vi "Dashboard Main.vi"() -> ()   [LabVIEW 2012]
uses:
  <vilib>/event_ctls.llb/eventvkey.ctl
  <vilib>/Utility/config.llb/Read Key (String).vi
  <vilib>/Utility/config.llb/Read Key (I32).vi
  <vilib>/Utility/config.llb/Write Key (String).vi
  <vilib>/Utility/config.llb/Write Key (I32).vi
  <vilib>/Utility/config.llb/NI_LVConfig.lvlib
panel:
  out "Battery Value":dbl(slide) scale=0.0..14.0 scale format="%#_2e"
  out "Battery":sgl(graph)
  in  "Camera Settings":T1={"Frate Rate"=30, "Compression"=30, "Size"=1} {"Frate Rate" scale=1.0..30.0; "Size" items=["640x480", "320x240", "160x120"]}
  out "Mode":T2(ring)=enum."Auto Disabled"
  out "Camera IP":string
  out "JS1 Z":dbl(slide) scale=-1.0..1.0 scale format="%#_2e"
  out "JS2 Z":dbl(slide) scale=-1.0..1.0 scale format="%#_2e"
  out "Joystick 1":cluster{"X":dbl, "Y":dbl}[](graph)
  out "Joystick 2":cluster{"X":dbl, "Y":dbl}[](graph)
  out "JS Buttons 1":T3
  out "JS Buttons 2":T3
  out "MotorSlide4":dbl(slide) scale=-1.0..1.0 scale format="%#_2e"
  out "MotorSlide3":dbl(slide) scale=-1.0..1.0 scale format="%#_2e"
  out "MotorSlide2":dbl(slide) scale=-1.0..1.0 scale format="%#_2e"
  out "MotorName3":string="Front Left"
  out "MotorName4":string="Front Right"
  out "MotorName1":string="Rear Left"
  out "MotorName2":string="Rear Right"
  out "MotorChart4":dbl(graph)
  out "MotorChart3":dbl(graph)
  out "MotorChart2":dbl(graph)
  out "MotorSlide1":dbl(slide) scale=-1.0..1.0 scale format="%#_2e"
  out "MotorChart1":dbl(graph)
  out "Robot IP":string
  in  "Dashboard Tab":T4(tab)
  in  "Disable Autonomous":bool
  out "Arm Hook Sensor":bool
  out "Arm Encoder":dbl(knob) scale=0.0..100.0
  in  "notes":string
  out "Right Hook Sensor":bool
  out "Left Hook Sensor":bool
  out "Encoder Set":bool
  out "Arm Limit":bool
  in  "Dev Notes":string
  in  "Robot Subsystems":enum32{"Drive", "Arm", "Sensors", "Hotkeys"}(tab)
  in  "X-Throttle":dbl(slide)=1.0 min=0.0 max=1.0 step=0.1 scale=0.0..1.0
  in  "Y-Throttle":dbl(slide)=1.0 min=0.0 max=1.0 step=0.1 scale=0.0..1.0
  out "Left Wheel Encoder":dbl
  out "Right Wheel Encoder":dbl
  in  "Override Limit":bool
  out "Right Ultrasonic PWM":dbl(slide) scale=0.0..100.0
  out "Gyro":dbl(knob) scale=-180.0..180.0
  out "Left Ultrasonic PWM":dbl(slide) scale=0.0..100.0
  out "Hotkey Step":dbl
  out "Arm Preset":dbl
  in  "Current Hotkey":string
  out "Hotkey Running?":bool
  in  "Sim":bool=TRUE
  in  "Slider":dbl(slide) scale=0.0..100.0 scale format="%#_3g"
  in  "On/Off":bool caption="Solenoid"
  in  "Test Name":u16(ring) items=["Select the test to run...", "Example Test", "-------------------------------", "List of tests is built in robot code.", "Replace with your own automated tests."]
  in  "Test Tree":string(tree)
  in  "Motor":cluster{"Value":dbl, "Enable":bool} {"Value" scale=-1.0..1.0 scale format="%#_3g"}
  out "Progress":T5 {"Test Progress" scale=0.0..100.0}
  in  "Rev/Fwd":cluster{"Forward":bool, "Reverse":bool}
  in  "Ring":u16(ring) items=["Auto", "Fixed indoor", "Fixed outdoor 1", "Fixed outdoor 2", "Fixed fluorescent 1", "Fixed fluorescent 2", "Hold current"]
  in  "Listbox":i32(listbox)
  in  "Viewer":T6(tab)
  out "Mbps":dbl format="%#.1g"
  in  "Enable":bool
  in  "DB Camera Config":bool
  out "Mbps":bool
  out "fps":dbl format="%#.1g"
  out "Image Error Message":string="Timeout in Camera Communications"
  out "Camera Image":T7(plugin-control)
  out "Buttons 1":cluster{"1":bool, "2":bool, "3":bool}
  out "Kinect 1":cluster{"X":dbl, "Y":dbl, "Z":dbl} {"X" scale=1.0..-1.0; "Y" scale=1.0..-1.0; "Z" scale=1.0..-1.0}
  out "Buttons 2":cluster{"1":bool, "2":bool, "3":bool}
  out "Kinect 2":cluster{"X":dbl, "Y":dbl, "Z":dbl} {"X" scale=1.0..-1.0; "Y" scale=1.0..-1.0; "Z" scale=1.0..-1.0}
  out "Version":string
  out "Skeleton Picture":picture
  out "Players":i8
  out "Tree":string(tree)
  # "Drive & Motors"
  # "Robot IP:"
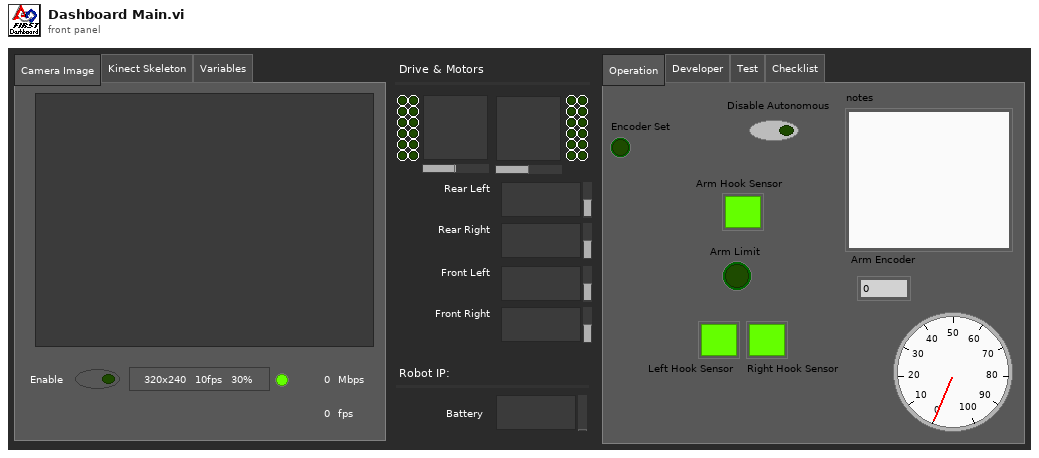
[diagram p1: front panel]
types:
  T1 = cluster{"Frate Rate":i32, "Compression":i32, "Size":u16}
  T2 = enum8{"Tele-Op Disabled", "Tele-Op Enabled", "Auto Disabled", "Auto Enabled", "Test Disabled", "Test Enabled", ""}
  T3 = cluster{bool, bool, bool, bool, bool, bool, bool, bool, bool, bool, bool, bool}
  T4 = enum32{"Operation", "Developer", "Test", "Checklist"}
  T5 = cluster{"Test Progress":u8, "Test Progress Text":string}
  T6 = enum32{"Camera Image", "Kinect Skeleton", "Variables"}
  T7 = typedef "IMAQ Image.ctl" = refnum<image>
  T8 = typedef "Image Type" = u32
  T9 = typedef "LVBoundsTypeDef.ctl" = cluster{"Width":u32, "Height":u32}
  T10 = typedef "SkeletonTrackState.ctl" = enum32{"NotTracked", "PositionOnly", "Tracked"}
  T11 = cluster{"TrackingState":u8[], "Position":cluster{"x":sgl, "y":sgl, "z":sgl}, cluster{"x":sgl, "y":sgl, "z":sgl, sgl}[], "TrackState":T10}
  T12 = cluster{cluster{"ScaledToPercentRange":dbl, "ScaledToPercentRange":dbl, "ScaledToPercentRange":dbl}, cluster{bool, bool, bool}}[]
  T13 = cluster{cluster{"ScaledToPercentRange":dbl, "ScaledToPercentRange":dbl, "ScaledToPercentRange":dbl}, cluster{bool, bool, bool}}
  T14 = cluster{"ScaledToPercentRange":dbl, "ScaledToPercentRange":dbl, "ScaledToPercentRange":dbl}
  T15 = typedef "LVRectTypeDef.ctl" = cluster{"Left":i16, "Top":i16, "Right":i16, "Bottom":i16}
  T16 = cluster{"Competition mode":bool, "Robot Link":bool, "Autonomous":bool, "Enabled":bool, "E-Stop":bool, "Simulated":bool, "TestMode":bool, "Docked Window":bool}
  T17 = cluster{"Boolean Array[0]":bool, "Boolean Array[1]":bool, "Boolean Array[2]":bool, "Boolean Array[3]":bool, "Boolean Array[4]":bool, "Boolean Array[5]":bool, "Boolean Array[6]":bool, "Boolean Array[7]":bool, "Boolean Array[8]":bool, "Boolean Array[9]":bool, "Boolean Array[10]":bool, "Boolean Array[11]":bool}
  T18 = typedef "NI_LVConfig.lvlib/Config Data RefNum.ctl" = refnum<k1>
  T19 = typedef "eventvkey.ctl" = enum16{"ASCII", "Enter", "Return", "Shift", "Ctrl", "Alt", "Cmd", "Opt", "Caps", "NumLock", "Clear", "Break", "Up", "Down", "Left", "Right", "Insert", "Delete", "Home", "End", "PageUp", "PageDown", "Escape", "Help", "Pause", "ScrollLock", "F1", "F2", "F3", "F4", "F5", "F6", "F7", "F8", "F9", "F10", "F11", "F12", "F13", "F14", "F15", "F16", "F17", "F18", "F19", "F20", "F21", "F22", "F23", "F24", "Play", "VolumeUp", "VolumeDown", "Mute", "Two Byte Char"}
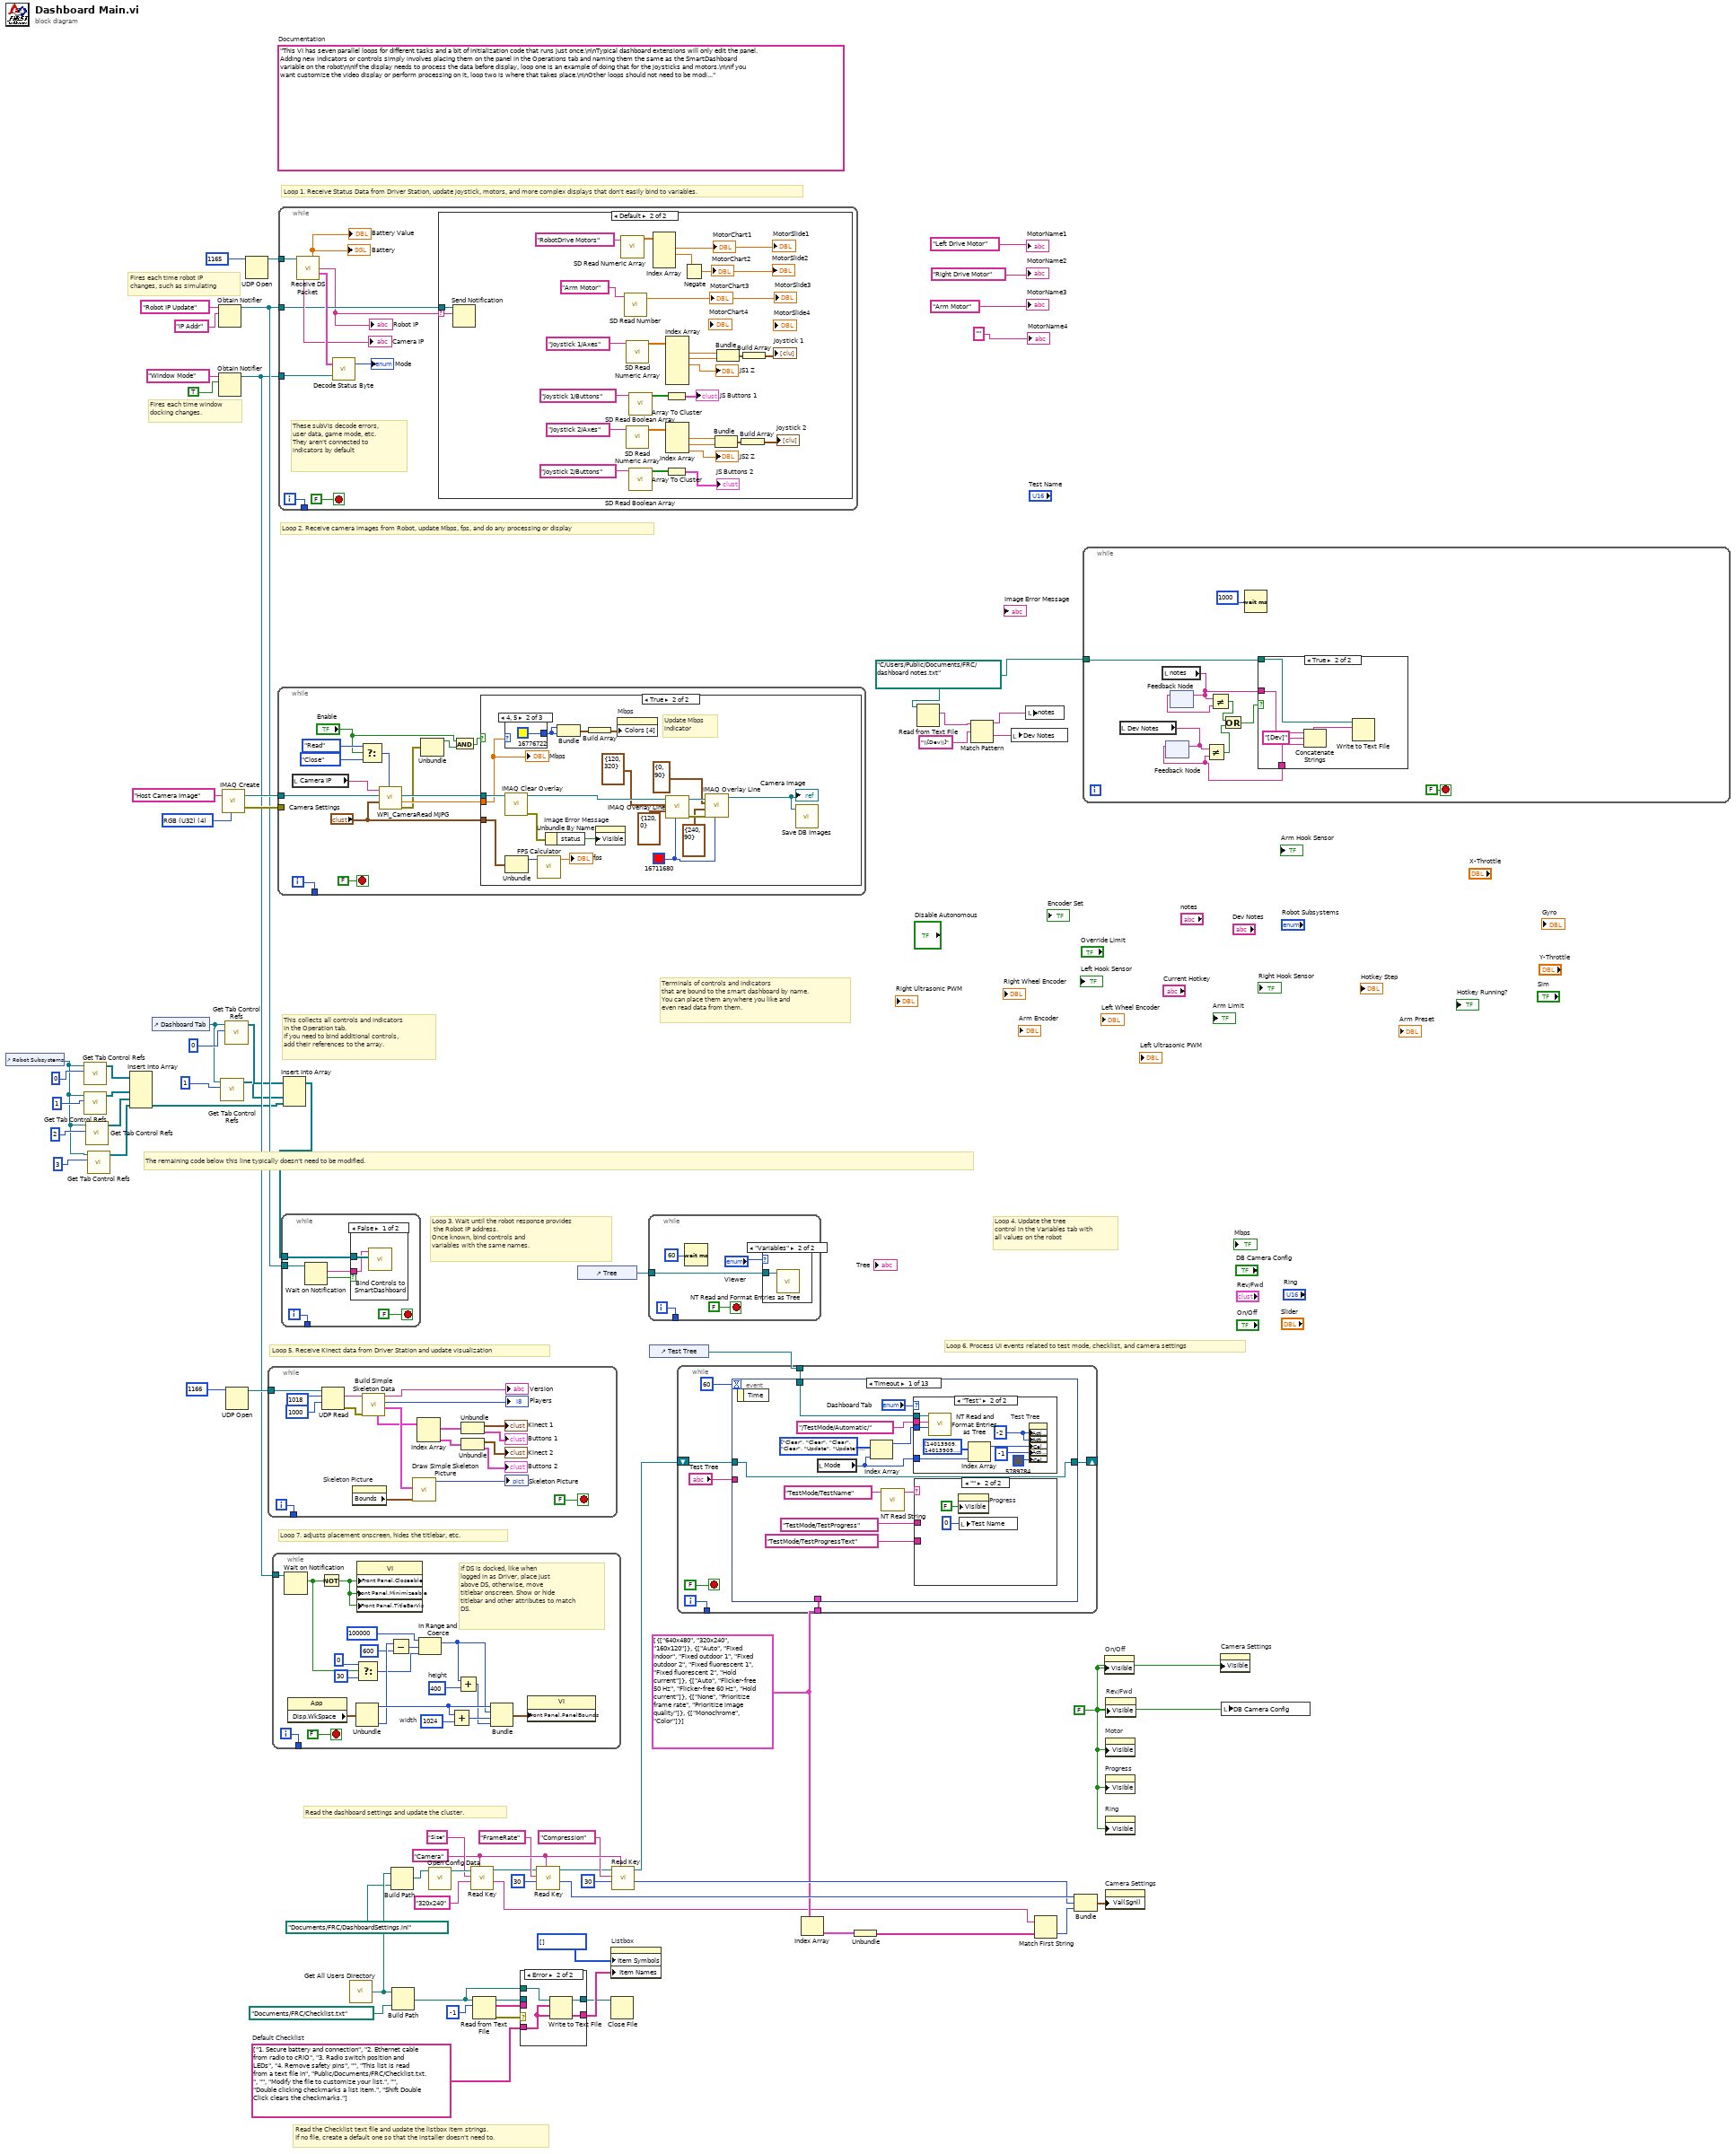
[diagram p0: block diagram]
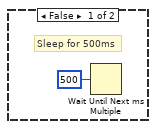
[diagram p4: hidden frame]
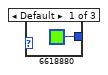
[diagram p5: hidden frame]
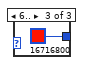
[diagram p6: hidden frame]
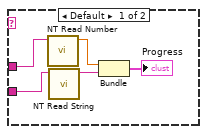
[diagram p9: hidden frame]
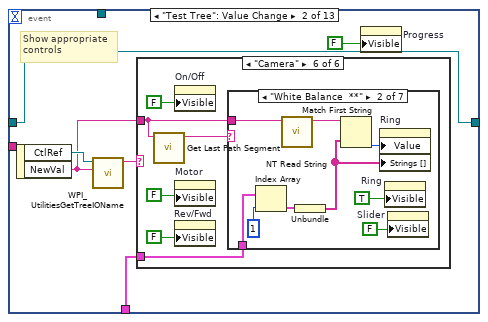
[diagram p10: hidden frame]
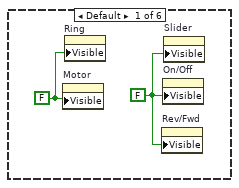
[diagram p11: hidden frame]
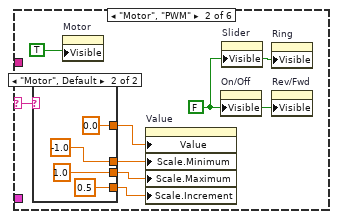
[diagram p12: hidden frame]
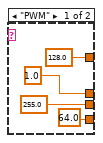
[diagram p13: hidden frame]
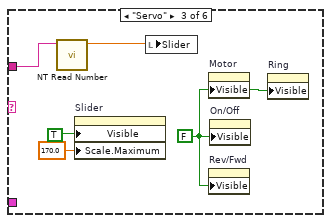
[diagram p14: hidden frame]
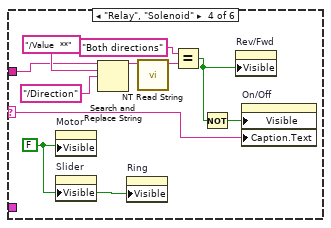
[diagram p15: hidden frame]
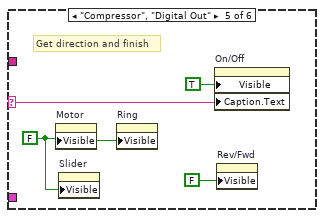
[diagram p16: hidden frame]
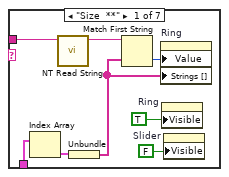
[diagram p17: hidden frame]
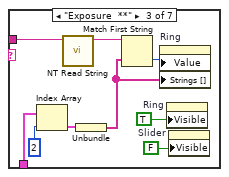
[diagram p18: hidden frame]
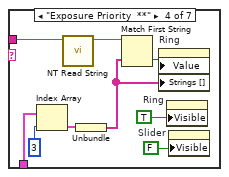
[diagram p19: hidden frame]
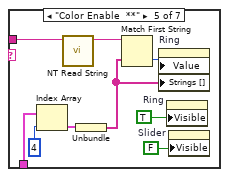
[diagram p20: hidden frame]
diagram:
  w15 = path "C:/Users/Public/Documents/FRC/dashboard notes.txt"
  w46 = "Camera"
  w38 = cluster{string[]}[] [{["640x480", "320x240", "160x120"]}, {["Auto", "Fixed indoor", "Fixed outdoor 1", "Fixed outdoor 2", "Fixed fluorescent 1", "Fixed fluorescent 2", "Hold current"]}, {["Auto", "Flicker-free 50 Hz", "Flicker-free 60 Hz", "Hold current"]}, {["None", "Prioritize frame rate", "Prioritize image quality"]}, {["Monochrome", "Color"]}]
  w54 = string[] ["1. Secure battery and connection", "2. Ethernet cable from radio to cRIO", "3. Radio switch position and LEDs", "4. Remove safety pins", "", "This list is read from a text file in", "Public/Documents/FRC/Checklist.txt.", "", "Modify the file to customize your list.", "", "Double clicking checkmarks a list item.", "Shift Double Click clears the checkmarks."]  # Default Checklist
  w52 = FALSE ("Visible")
  (unwired) "This VI has seven parallel loops for different tasks and a bit of initialization code that runs just once.\n\nTypical dashboard extensions will only edit the panel. Adding new indicators or controls simply involves placing them on the panel in the Operations tab and naming them the same as the SmartDashboard variable on the robot\n\nIf the display needs to process the data before display, loop one is an example of doing that for the joysticks and motors.\n\nIf you want customize the video display or perform processing on it, loop two is where that takes place.\n\nOther loops should not need to be modified. They are pretty standard, and document the task they perform."  # Documentation
  w72 = T8 4 items=["Grayscale (U8)", "Grayscale (I16)", "Grayscale (SGL)", "Complex (CSG)", "RGB (U32)", "HSL (U32)", "RGB (U64)"] ("Image Type")
  # "Fires each time robot IP\nchanges, such as simulating"
  # "Fires each time window\ndocking changes."
  # "Read the Checklist text file and update the listbox item strings.\nIf no file, create a default one so that the installer doesn't need to."
  # "This collects all controls and indicators\nin the Operation tab.\nIf you need to bind additional controls,\nadd their references to the array."
  # "The remaining code below this line typically doesn't need to be modified."
  # "Loop 6. Process UI events related to test mode, checklist, and camera settings"
  # "Read the dashboard settings and update the cluster."
  # "Terminals of controls and indicators\nthat are bound to the smart dashboard by name.\nYou can place them anywhere you like and\neven read data from them."
  # "Loop 4. Update the tree\ncontrol in the Variables tab with\nall values on the robot"
  # "Loop 3. Wait until the robot response provides\n the Robot IP address.\nOnce known, bind controls and\nvariables with the same names."
  # "Loop 5. Receive Kinect data from Driver Station and update visualization"
  # "Loop 7. adjusts placement onscreen, hides the titlebar, etc."
  # "Loop 1. Receive Status Data from Driver Station, update joystick, motors, and more complex displays that don't easily bind to variables."
  # "Loop 2. Receive camera images from Robot, update Mbps, fps, and do any processing or display"
  n1 = control-ref of="Robot Subsystems"() -> (w4:refnum<vi>)
  n2 = call <vilib>:"Get Tab Control Refs.vi"("Page Index"=0, "TabControl in"=w4) -> ("ControlsOnPage"=w8:refnum<vi>[])  [unwired: 9 in]
  n3 = call <vilib>:"Get Tab Control Refs.vi"("Page Index"=1, "TabControl in"=w4) -> ("ControlsOnPage"=w3:refnum<vi>[])  [unwired: 9 in]
  n4 = call <vilib>:"Get Tab Control Refs.vi"("Page Index"=2, "TabControl in"=w4) -> ("ControlsOnPage"=w2:refnum<vi>[])  [unwired: 9 in]
  n5 = call <vilib>:"Get Tab Control Refs.vi"("Page Index"=3, "TabControl in"=w4) -> ("ControlsOnPage"=w1:refnum<vi>[])  [unwired: 9 in]
  n6 = Insert Into Array(array=w8, new element #1=w3, new element #2=w2, new element #3=w1) -> (w9:refnum<vi>[])  [unwired: 1 in]
  n7 = control-ref of="Dashboard Tab"() -> (w19:refnum<vi>)
  n8 = Obtain Notifier(name (unnamed)="Robot IP Update", notification data type="IP Addr" ("name (unnamed)")) -> (notifier out=w64:refnum<notifier>)  [unwired: 2 in, 2 out]
  n9 = Obtain Notifier(name (unnamed)="Window Mode", notification data type=TRUE) -> (notifier out=w58:refnum<notifier>)  [unwired: 2 in, 2 out]
  n10 = call <vilib>:"Get Tab Control Refs.vi"("Page Index"=1, "TabControl in"=w19) -> ("ControlsOnPage"=w17:refnum<vi>[])  [unwired: 9 in]
  n11 = call "IMAQ Create"("Image Name"="Host Camera Image", "Image Type"=w72) -> ("New Image"=w70:T7, "error out"=w69:errorcluster)  [unwired: 2 in, 1 out]
  n12 = call <vilib>:"Get Tab Control Refs.vi"("Page Index"=0, "TabControl in"=w19) -> ("ControlsOnPage"=w21:refnum<vi>[])  [unwired: 9 in]
  n13 = UDP Open(11:u16 1166 ("port")) -> (port=w67:refnum<k16>)  [unwired: 2 in, 4 out]
  n14 = UDP Open(11:u16 1165 ("port")) -> (port=w73:refnum<k16>)  [unwired: 2 in, 4 out]
  n15 = while {
    tunnel: w67 -> [w91]
    tunnel: [w76] -> _
    i -> [w76]
    stop <- FALSE stop-if-true
    n16 = UDP Read(connection ID=w91, max size (548)=1018 ("bytes to read"), timeout ms (25000)=1000) -> (data out=w85:string, error out=w75:errorcluster)  [unwired: 1 in, 3 out]
    n17 = property on="Skeleton Picture" class="Pict"() -> ("Bounds"=w87:T9)  [unwired: 2 in, 2 out]
    n18 = call "Build Simple Skeleton Data.vi"("error in (no error)"=w75, "data in"=w85) -> ("Skeleton Data"=w86:T11, "NumPlayers"=→"Players":i8, "Version String"=→"Version":string, "Simple Joystick Info"=w83:T12)  [unwired: 5 in, 1 out]
    n19 = call "Draw Simple Skeleton Picture.vi"("Bounds"=w87, "Simple Skeleton"=w86) -> ("new picture out"=→"Skeleton Picture":picture)  [unwired: 9 in]
    n20 = Index Array(array=w83) -> (element #1=w82:T13, element #2=w81:T13)  [unwired: 2 in]
    n21 = Unbundle(w82) -> (→"Kinect 1":T14, →"Buttons 1":cluster{bool, bool, bool})
    n22 = Unbundle(w81) -> (→"Kinect 2":T14, →"Buttons 2":cluster{bool, bool, bool})
  }
  n23 = while {
    tunnel: w58 -> [w112]
    tunnel: [w110] -> _
    i -> [w110]
    stop <- FALSE stop-if-true
    w102 = 1024  # width
    w105 = 400  # height
    # "If DS is docked, like when\nlogged in as Driver, place just\nabove DS, otherwise, move\ntitlebar onscreen. Show or hide\ntitlebar and other attributes to match\nDS."
    n24 = Wait on Notification(notifier=w112) -> (notification=w97:bool)  [unwired: 3 in, 3 out]
    n25 = property class="App"() -> ("Disp.WkSpace"=w108:T15)  [unwired: 2 in, 2 out]
    n26 = Not(x=w97) -> (.not. x?=w111:bool)
    n27 = Unbundle(w108) -> ("Left"=w106:i16, "Bottom"=w103:i16)  [unwired: 2 out]
    n28 = Select(t=0, s=w97, f=30) -> (s? t:f=w96:i32)
    n29 = property class="VI"("Front Panel.Closeable"=w111, "Front Panel.Minimizeable"=w111, "Front Panel.TitleBarVis"=w111) -> ()  [unwired: 2 in, 2 out]
    n30 = Subtract(x=w103, y=600) -> (x-y=w100:i32)
    n31 = In Range and Coerce(upper limit=100000, x=w100, lower limit=w96) -> (coerced(x)=w94:i32)  [unwired: 1 out]
    n32 = Add(x=w106, y=w102) -> (x+y=w107:i32)
    n33 = Add(x=w94, y=w105) -> (x+y=w104:i32)
    n34 = Bundle("Left"=w106, w94, w107, w104) -> (w109:cluster{"Left":i16, i32, i32, i32})  [unwired: 1 out]
    n35 = property class="VI"("Front Panel.PanelBounds"=w109) -> ()  [unwired: 2 in, 2 out]
  }
  n36 = while {
    tunnel: w70 -> [w123]
    tunnel: w69 -> [_]
    tunnel: [w126] -> _
    i -> [w126]
    stop <- FALSE stop-if-true
    n37 = local read "Camera IP"() -> (w125:string)
    n38 = Select(t=enum16{"Read", "Reopen", "Close"}."Read" ("Operation"), s="Enable", f=enum16{"Read", "Reopen", "Close"}."Close" ("Operation")) -> (s? t:f=w118:enum16{"Read", "Reopen", "Close"})
    n39 = call <vilib>:"WPI_CameraRead MJPG.vi"("Operation"=w118, "Camera Settings"="Camera Settings", "Image"=w123, "address"=w125) -> ("error out"=w117:errorcluster, "Bandwidth (kbps)"=w121:dbl, "Image Out"=w122:T7)  [unwired: 5 in]
    n40 = Unbundle(w117) -> ("status"=w114:bool)  [unwired: 2 out]
    n41 = And(x="Enable", y=w114) -> (x .and. y?=w116:bool)
    n42 = case shown="True" w116 {
      tunnel: "Camera Settings" -> [_ w139]
      tunnel: w122 -> [_ w142]
      tunnel: w121 -> [_ w141]
      frame False {
        # "Sleep for 500ms"
        n43 = Wait Until Next ms Multiple(millisecond multiple=u32 500) -> ()  [unwired: 1 out]
      }
      frame True {
        w129 = u32 16711680 ("Color Box")
        # "Update Mbps\nindicator"
        n44 = call "IMAQ Clear Overlay"("Image"=w142) -> ("error out"=w146:errorcluster, "Image Out"=w137:T7)  [unwired: 2 in, 7 out]
        n45 = case shown="4, 5" w141 {
          tunnel: [u32 6618880 ("Color Box") u32 16776722 ("Color Box") u32 16716800 ("Color Box")] -> w143
          frame Default {
          }
          frame 4, 5 {
          }
          frame 6.. {
          }
        }
        n46 = Unbundle(w139) -> ("Frate Rate"=w138:i32)  [unwired: 2 out]
        n47 = call "FPS Calculator.vi"("Average Count"=w138) -> ("fps"=→"fps":dbl)  [unwired: 10 in]
        n48 = Unbundle By Name(w146) -> ("status"=w147:bool)
        n49 = Bundle("Color Box"=w143, "Color Box"=w143) -> (w145:cluster{"Color Box":u32, "Color Box":u32})  [unwired: 1 out]
        n50 = Build Array(w145) -> (w144:cluster{"Color Box":u32, "Color Box":u32}[])
        n51 = property on="Image Error Message" class="Str"("Visible"=w147) -> ()  [unwired: 2 in, 2 out]
        n52 = property on="Mbps" class="Bool (strict)"("Colors [4]"=w144) -> ()  [unwired: 2 in, 2 out]
        n53 = call "IMAQ Overlay Line"("Color"=w129, "End Point"=cluster{"X":i32, "Y":i32} {"X"=120, "Y"=0} ("Start Point"), "Start Point"=cluster{"X":i32, "Y":i32} {"X"=120, "Y"=320}, "Image"=w137) -> ("error out"=w134:errorcluster, "Image Out"=w133:T7)  [unwired: 6 in]
        n54 = call "IMAQ Overlay Line"("Color"=w129, "error in (no error)"=w134, "End Point"=cluster{"X":i32, "Y":i32} {"X"=240, "Y"=90} ("Start Point"), "Start Point"=cluster{"X":i32, "Y":i32} {"X"=0, "Y"=90}, "Image"=w133) -> ("Image Out"=w132:T7)  [unwired: 5 in, 1 out]
        "Camera Image" <- w132
        n55 = call "Save DB Images.vi"("Image"=w132) -> ()  [unwired: 2 in, 1 out]
        "Mbps" <- w141
      }
    }
  }
  n56 = while {
    tunnel: w73 -> [w158]
    tunnel: w64 -> [w152]
    tunnel: w58 -> [w156]
    tunnel: [w153] -> _
    i -> [w153]
    stop <- FALSE stop-if-true
    # "These subVIs decode errors, user data, game mode, etc.\nThey aren't connected to indicators by default"
    n57 = call "Receive DS Packet.vi"("Recv Socket"=w158) -> ("Battery"=→"Battery" →"Battery Value":sgl, "Robot IP Address"=w151:string, "Status"=w159:T16, "Camera IP Address"=→"Camera IP":string)  [unwired: 1 in, 10 out]
    "Robot IP" <- w151
    n58 = call "Decode Status Byte.vi"("Window Mode Notifier"=w156, "Status"=w159) -> ("Mode"=→"Mode":T2)  [unwired: 1 out]
    n59 = case shown="Default" w151 {
      selector: w151 -> [_ w166]
      tunnel: w152 -> [_ w167]
      frame "0.0.0.0" {
        # "Robot not responding, don't poll the variables"
      }
      frame Default {
        n60 = Send Notification(notification=w166, notifier=w167) -> ()  [unwired: 1 in, 2 out]
        n61 = call <vilib>:"SD Read Numeric Array.vi"("Name"="RobotDrive Motors") -> ("Numeric Array"=w186:dbl[])  [unwired: 8 in, 2 out]
        n62 = call <vilib>:"SD Read Number.vi"("Name"="Arm Motor") -> ("Numeric"=→"MotorChart3" →"MotorSlide3":dbl)  [unwired: 8 in, 2 out]
        n63 = call <vilib>:"SD Read Numeric Array.vi"("Name"="Joystick 1/Axes") -> ("Numeric Array"=w182:dbl[])  [unwired: 8 in, 2 out]
        n64 = call <vilib>:"SD Read Numeric Array.vi"("Name"="Joystick 2/Axes") -> ("Numeric Array"=w177:dbl[])  [unwired: 8 in, 2 out]
        n65 = call <vilib>:"SD Read Boolean Array.vi"("Name"="Joystick 1/Buttons") -> ("Boolean Array"=w184:bool[])  [unwired: 8 in, 2 out]
        n66 = call <vilib>:"SD Read Boolean Array.vi"("Name"="Joystick 2/Buttons") -> ("Boolean Array"=w176:bool[])  [unwired: 8 in, 2 out]
        n67 = Index Array(array=w186) -> (element #1=→"MotorChart1" →"MotorSlide1":dbl, element #2=w162:dbl)  [unwired: 4 in, 2 out]
        n68 = Array To Cluster(array=w184) -> (cluster=→"JS Buttons 1":T17)
        n69 = Array To Cluster(array=w176) -> (cluster=→"JS Buttons 2":T17)
        n70 = Index Array(array=w182) -> (element #1=w180:dbl, element #2=w181:dbl, element #3=→"JS1 Z":dbl)  [unwired: 6 in, 3 out]
        n71 = Index Array(array=w177) -> (element #1=w172:dbl, element #2=w171:dbl, element #3=→"JS2 Z":dbl)  [unwired: 3 in]
        n72 = Negate(x=w162) -> (-x=→"MotorSlide2" →"MotorChart2":dbl)
        n73 = Bundle("Numeric"=w172, "Numeric"=w171) -> (w173:cluster{"Numeric":dbl, "Numeric":dbl})  [unwired: 1 in]
        n74 = Bundle("Numeric"=w180, "Numeric"=w181) -> (w179:cluster{"Numeric":dbl, "Numeric":dbl})  [unwired: 1 in]
        n75 = Build Array(w173) -> (→"Joystick 2":cluster{"Numeric":dbl, "Numeric":dbl}[])
        n76 = Build Array(w179) -> (→"Joystick 1":cluster{"Numeric":dbl, "Numeric":dbl}[])
      }
    }
  }
  n77 = Insert Into Array(array=w21, new element #1=w17, new element #2=w9) -> (w20:refnum<vi>[])  [unwired: 1 in]
  n78 = while {
    tunnel: w20 -> [w195]
    tunnel: w64 -> [w192]
    tunnel: [w190] -> _
    i -> [w190]
    stop <- FALSE stop-if-true
    n79 = Wait on Notification(notifier=w192) -> (notification=w191:string, timed out?=w193:bool)  [unwired: 3 in, 2 out]
    n80 = case shown="False" w193 {
      tunnel: w195 -> [w197 _]
      tunnel: w191 -> [w196 _]
      frame False {
        n81 = call <vilib>:"Bind Controls to SmartDashboard.vi"("Bound Control Refs"=w197, "Server IP Address"=w196) -> ()  [unwired: 10 in]
      }
      frame True {
      }
    }
  }
  n82 = call "Get All Users Directory.vi"() -> ("All User Path"=w51:path)
  n83 = Build Path(base path=w51, name or relative path=path "Documents/FRC/DashboardSettings.ini") -> (appended path=w50:path)
  n84 = Build Path(base path=w51, name or relative path=path "Documents/FRC/Checklist.txt") -> (appended path=w55:path)
  n85 = call <vilib>:"Open Config Data.vi"("configuration file path"=w50) -> ("refnum"=w49:T18)  [unwired: 8 in, 2 out]
  n86 = call-poly <vilib>:"Read Key.vi"("section"=w46, "default value"="320x240", "key"="Size", "refnum"=w49) -> ("value"=w36:string, "refnum out"=w31:T18)  [unwired: 2 in, 4 out]
  n87 = Read from Text File(file (use dialog)=w55, count=-1 ("timeout ms (25000)")) -> (refnum out=w33:refnum<file>, text=w56:string[], error out=w57:errorcluster)  [unwired: 2 in, 1 out]
  n88 = case shown="Error" w57 {
    tunnel: w56 -> [w199 _]
    tunnel: [w199 w201] -> w53
    tunnel: w54 -> [_ w201]
    tunnel: w55 -> [_ w202]
    tunnel: [w198 w200] -> w32
    tunnel: w33 -> [w198 _]
    frame No Error {
    }
    frame Error {
      n89 = Write to Text File(file (use dialog)=w202, text=w201) -> (refnum out=w200:refnum<file>)  [unwired: 2 in, 2 out]
    }
  }
  n90 = call-poly <vilib>:"Read Key.vi"("section"=w46, "default value"=30, "key"="FrameRate", "refnum"=w31) -> ("value"=w41:i32, "refnum out"=w30:T18)  [unwired: 1 in, 5 out]
  n91 = control-ref of="Tree"() -> (w27:refnum<vi>)
  n92 = property on="Listbox" class="LstBox (strict)"("Item Symbols"=i32[] [], "Item Names"=w53) -> ()  [unwired: 2 in, 2 out]
  n93 = Close File(refnum=w32) -> ()  [unwired: 1 in, 2 out]
  n94 = call-poly <vilib>:"Read Key.vi"("section"=w46, "default value"=30, "key"="Compression", "refnum"=w30) -> ("value"=w40:i32, "refnum out"=w28:T18)  [unwired: 1 in, 5 out]
  n95 = while {
    tunnel: [w204] -> _
    tunnel: w27 -> [w203]
    i -> [w204]
    stop <- FALSE stop-if-true
    n96 = Wait (ms)(milliseconds to wait=u32 60) -> ()  [unwired: 1 out]
    n97 = case shown="\"Variables\"" "Viewer" {
      tunnel: w203 -> [_ w208]
      frame Default {
      }
      frame "Variables" {
        n98 = call <vilib>:"NT Read and Format Entries as Tree.vi"("Tree Refnum"=w208) -> ()  [unwired: 9 in, 2 out]
      }
    }
  }
  n99 = control-ref of="Test Tree"() -> (w26:refnum<vi>)
  n100 = while {
    tunnel: w38 -> [w213]
    shift-right: [w212] -> _
    shift-left: w28 -> [w211]
    tunnel: [w210] -> _
    tunnel: w26 -> [w209]
    i -> [w210]
    stop <- FALSE stop-if-true
    n101 = event shown="[0] Timeout" {
      selector: _ -> [_ _ _ _ _ _ _ _ _ _ _ _ _]
      dyn-events: _ -> [_ _ _ _ _ _ _ _ _ _ _ _ _]
      timeout: u32 60 ("milliseconds to wait") -> [_ _ _ _ _ _ _ _ _ _ _ _ _]
      tunnel: w209 -> [w223 _ _ _ _ _ _ _ _ _ _ _ _]
      tunnel: "Test Tree" -> [_ _ _ _ _ _ _ _ w417 w425 w427 w431 w439]
      tunnel: w213 -> [_ w245 _ _ _ _ w381 w411 _ _ _ _ _]
      tunnel: [w217 w244 _ w347 w355 w367 w380 w404 w416 w423 w426 w430 w438] -> w212
      tunnel: w211 -> [w217 w244 _ w347 w355 w367 w379 w404 w416 w423 w426 w430 w438]
      event Timeout {
        w222 = enum16{"Update", "Clear"}[] [enum."Clear", enum."Clear", enum."Clear", enum."Clear", enum."Update", enum."Update", enum."Clear"] items=["Update", "Clear"]
        n102 = event-data() -> ()  [unwired: 1 in, 1 out]
        n103 = local read "Mode"() -> (w220:T2)
        n104 = Index Array(array=w222, index=w220) -> (element=w221:enum16{"Update", "Clear"})
        n105 = call <vilib>:"NT Read String.vi"("Name"="TestMode/TestName") -> ("String"=w226:string)  [unwired: 9 in, 1 out]
        n106 = case shown="\"Test\"" "Dashboard Tab" {
          tunnel: w223 -> [_ w236]
          tunnel: "/TestMode/Automatic/" ("Name Pattern") -> [_ w235]
          tunnel: w221 -> [_ w234]
          tunnel: w220 -> [_ w232]
          frame "Operation", Default {
          }
          frame "Test" {
            w231 = -2 ("Active Item:Row Number")
            n107 = call <vilib>:"NT Read and Format Entries as Tree.vi"("Operation"=w234, "Name Pattern"=w235, "Tree Refnum"=w236) -> ()  [unwired: 7 in, 2 out]
            n108 = Index Array(array=u32[] [14013909, 14013909, 14013909, 14013909, 14013909, 16777215, 14013909], index=w232) -> (element=w230:u32)
            n109 = property on="Test Tree" class="Tree (strict)"("Active Item Row Number"=w231, "ActiveColNum"=w231, "CellBG"=w230, "Active Item Row Number"=-1 ("Active Item:Row Number"), "CellBG"=u32 5789784 ("Color Box")) -> ()  [unwired: 2 in, 2 out]
          }
        }
        n110 = case shown="\"\"" w226 {
          tunnel: "TestMode/TestProgress" ("Name") -> [w238 _]
          tunnel: "TestMode/TestProgressText" ("Name") -> [w237 _]
          frame Default {
            n111 = call <vilib>:"NT Read Number.vi"("Name"=w238) -> ("Numeric"=w239:dbl)  [unwired: 9 in, 1 out]
            n112 = call <vilib>:"NT Read String.vi"("Name"=w237) -> ("String"=w240:string)  [unwired: 9 in, 1 out]
            n113 = Bundle("Numeric"=w239, "String"=w240) -> (→"Progress":cluster{"Numeric":dbl, "String":string})  [unwired: 1 in]
          }
          frame "" {
            n114 = property on="Progress" class="Clust (strict)"("Visible"=FALSE) -> ()  [unwired: 2 in, 2 out]
            n115 = local write "Test Name"(u16 0) -> ()
          }
        }
      }
      event "Test Tree": Value Change {
        # "Show appropriate\ncontrols"
        n116 = event-data() -> ("CtlRef"=w248:refnum<vi>, "NewVal"=w246:string)  [unwired: 1 in]
        n117 = call <vilib>:"WPI_UtilitiesGetTreeIOName.vi"("NewVal"=w246, "TreeControl in"=w248) -> ("I/O Name"=w249:string)  [unwired: 9 in]
        n118 = case shown="\"Camera\"" w249 {
          selector: w249 -> [_ w256 _ w274 w283 _]
          tunnel: w246 -> [_ _ w271 w273 _ w290]
          tunnel: w245 -> [_ _ _ _ _ w289]
          frame Default {
            w251 = FALSE ("Visible")
            w250 = FALSE ("Visible")
            n119 = property on="Motor" class="Clust (strict)"("Visible"=w250) -> ()  [unwired: 2 in, 2 out]
            n120 = property on="Ring" class="Ring (strict)"("Visible"=w250) -> ()  [unwired: 2 in, 2 out]
            n121 = property on="Rev/Fwd" class="Clust (strict)"("Visible"=w251) -> ()  [unwired: 2 in, 2 out]
            n122 = property on="On/Off" class="Bool (strict)"("Visible"=w251) -> ()  [unwired: 2 in, 2 out]
            n123 = property on="Slider" class="Slide (strict)"("Visible"=w251) -> ()  [unwired: 2 in, 2 out]
          }
          frame "Motor", "PWM" {
            w257 = FALSE ("Visible")
            n124 = case shown="\"Motor\", Default" w256 {
              tunnel: [1.0 ("Value") -1.0 ("Value")] -> w255
              tunnel: [255.0 ("Value") 1.0 ("Value")] -> w254
              tunnel: [128.0 ("Value") 0.0 ("Value")] -> w253
              tunnel: [64.0 ("Value") 0.5 ("Value")] -> w252
              frame "PWM" {
              }
              frame "Motor", Default {
              }
            }
            n125 = property on="Motor" class="Clust (strict)"("Visible"=TRUE) -> ()  [unwired: 2 in, 2 out]
            n126 = property on="Value" class="Slide (strict)"("Value"=w253, "Scale.Minimum"=w255, "Scale.Maximum"=w254, "Scale.Increment"=w252) -> ()  [unwired: 2 in, 2 out]
            n127 = property on="On/Off" class="Bool (strict)"("Visible"=w257) -> ()  [unwired: 2 in, 2 out]
            n128 = property on="Slider" class="Slide (strict)"("Visible"=w257) -> ()  [unwired: 2 in, 2 out]
            n129 = property on="Ring" class="Ring (strict)"("Visible"=w257) -> ()  [unwired: 2 in, 2 out]
            n130 = property on="Rev/Fwd" class="Clust (strict)"("Visible"=w257) -> ()  [unwired: 2 in, 2 out]
          }
          frame "Servo" {
            w269 = FALSE ("Visible")
            n131 = call <vilib>:"NT Read Number.vi"("Name"=w271) -> ("Numeric"=w270:dbl)  [unwired: 9 in, 1 out]
            n132 = property on="Slider" class="Slide (strict)"("Visible"=TRUE, "Scale.Maximum"=170.0 ("Scale.Range:Maximum")) -> ()  [unwired: 2 in, 2 out]
            n133 = local write "Slider"(w270) -> ()
            n134 = property on="Motor" class="Clust (strict)"("Visible"=w269) -> ()  [unwired: 2 in, 2 out]
            n135 = property on="Rev/Fwd" class="Clust (strict)"("Visible"=w269) -> ()  [unwired: 2 in, 2 out]
            n136 = property on="On/Off" class="Bool (strict)"("Visible"=w269) -> ()  [unwired: 2 in, 2 out]
            n137 = property on="Ring" class="Ring (strict)"("Visible"=w269) -> ()  [unwired: 2 in, 2 out]
          }
          frame "Relay", "Solenoid" {
            w272 = FALSE ("Visible")
            n138 = property on="Motor" class="Clust (strict)"("Visible"=w272) -> ()  [unwired: 2 in, 2 out]
            n139 = property on="Slider" class="Slide (strict)"("Visible"=w272) -> ()  [unwired: 2 in, 2 out]
            n140 = Search and Replace String(input string=w273, search string="/Value  **", replace string="/Direction") -> (result string=w279:string)  [unwired: 5 in, 3 out]
            n141 = property on="Ring" class="Ring (strict)"("Visible"=w272) -> ()  [unwired: 2 in, 2 out]
            n142 = call <vilib>:"NT Read String.vi"("Name"=w279) -> ("String"=w277:string)  [unwired: 9 in, 1 out]
            n143 = Equal?(x="Both directions", y=w277) -> (x = y?=w275:bool)
            n144 = Not(x=w275) -> (.not. x?=w276:bool)
            n145 = property on="Rev/Fwd" class="Clust (strict)"("Visible"=w275) -> ()  [unwired: 2 in, 2 out]
            n146 = property on="On/Off" class="Bool (strict)"("Visible"=w276, "Caption.Text"=w274) -> ()  [unwired: 2 in, 2 out]
          }
          frame "Compressor", "Digital Out" {
            w282 = FALSE ("Visible")
            # "Get direction and finish"
            n147 = property on="Motor" class="Clust (strict)"("Visible"=w282) -> ()  [unwired: 2 in, 2 out]
            n148 = property on="Slider" class="Slide (strict)"("Visible"=w282) -> ()  [unwired: 2 in, 2 out]
            n149 = property on="Ring" class="Ring (strict)"("Visible"=w282) -> ()  [unwired: 2 in, 2 out]
            n150 = property on="On/Off" class="Bool (strict)"("Visible"=TRUE, "Caption.Text"=w283) -> ()  [unwired: 2 in, 2 out]
            n151 = property on="Rev/Fwd" class="Clust (strict)"("Visible"=FALSE) -> ()  [unwired: 2 in, 2 out]
          }
          frame "Camera" {
            n152 = call <vilib>:"Get Last Path Segment.vi"("String in"=w290) -> ("String out"=w291:string)  [unwired: 10 in]
            n153 = property on="On/Off" class="Bool (strict)"("Visible"=FALSE) -> ()  [unwired: 2 in, 2 out]
            n154 = property on="Motor" class="Clust (strict)"("Visible"=FALSE) -> ()  [unwired: 2 in, 2 out]
            n155 = property on="Rev/Fwd" class="Clust (strict)"("Visible"=FALSE) -> ()  [unwired: 2 in, 2 out]
            n156 = case shown="\"White Balance  **\"" w291 {
              tunnel: w290 -> [w297 w306 w315 w324 w333 _ w339]
              tunnel: w289 -> [w295 w303 w312 w321 w330 _ _]
              frame "Size  **" {
                n157 = Index Array(array=w295) -> (element=w294:cluster{string[]})  [unwired: 1 in]
                n158 = call <vilib>:"NT Read String.vi"("Name"=w297) -> ("String"=w296:string)  [unwired: 9 in, 1 out]
                n159 = Unbundle(w294) -> (w292:string[])
                n160 = Match First String(2:w292, 3:w296) -> (0:w293:i32)  [unwired: 1 out]
                n161 = property on="Ring" class="Ring (strict)"("Value"=w293, "Strings []"=w292) -> ()  [unwired: 2 in, 2 out]
                n162 = property on="Ring" class="Ring (strict)"("Visible"=TRUE) -> ()  [unwired: 2 in, 2 out]
                n163 = property on="Slider" class="Slide (strict)"("Visible"=FALSE) -> ()  [unwired: 2 in, 2 out]
              }
              frame "White Balance  **" {
                n164 = Index Array(array=w303, index=1) -> (element=w304:cluster{string[]})
                n165 = call <vilib>:"NT Read String.vi"("Name"=w306) -> ("String"=w305:string)  [unwired: 9 in, 1 out]
                n166 = Unbundle(w304) -> (w301:string[])
                n167 = Match First String(2:w301, 3:w305) -> (0:w300:i32)  [unwired: 1 out]
                n168 = property on="Ring" class="Ring (strict)"("Value"=w300, "Strings []"=w301) -> ()  [unwired: 2 in, 2 out]
                n169 = property on="Ring" class="Ring (strict)"("Visible"=TRUE) -> ()  [unwired: 2 in, 2 out]
                n170 = property on="Slider" class="Slide (strict)"("Visible"=FALSE) -> ()  [unwired: 2 in, 2 out]
              }
              frame "Exposure  **" {
                n171 = Index Array(array=w312, index=2) -> (element=w313:cluster{string[]})
                n172 = call <vilib>:"NT Read String.vi"("Name"=w315) -> ("String"=w314:string)  [unwired: 9 in, 1 out]
                n173 = Unbundle(w313) -> (w309:string[])
                n174 = Match First String(2:w309, 3:w314) -> (0:w310:i32)  [unwired: 1 out]
                n175 = property on="Ring" class="Ring (strict)"("Value"=w310, "Strings []"=w309) -> ()  [unwired: 2 in, 2 out]
                n176 = property on="Ring" class="Ring (strict)"("Visible"=TRUE) -> ()  [unwired: 2 in, 2 out]
                n177 = property on="Slider" class="Slide (strict)"("Visible"=FALSE) -> ()  [unwired: 2 in, 2 out]
              }
              frame "Exposure Priority  **" {
                n178 = Index Array(array=w321, index=3) -> (element=w322:cluster{string[]})
                n179 = call <vilib>:"NT Read String.vi"("Name"=w324) -> ("String"=w323:string)  [unwired: 9 in, 1 out]
                n180 = Unbundle(w322) -> (w318:string[])
                n181 = Match First String(2:w318, 3:w323) -> (0:w319:i32)  [unwired: 1 out]
                n182 = property on="Ring" class="Ring (strict)"("Value"=w319, "Strings []"=w318) -> ()  [unwired: 2 in, 2 out]
                n183 = property on="Ring" class="Ring (strict)"("Visible"=TRUE) -> ()  [unwired: 2 in, 2 out]
                n184 = property on="Slider" class="Slide (strict)"("Visible"=FALSE) -> ()  [unwired: 2 in, 2 out]
              }
              frame "Color Enable  **" {
                n185 = Index Array(array=w330, index=4) -> (element=w331:cluster{string[]})
                n186 = call <vilib>:"NT Read String.vi"("Name"=w333) -> ("String"=w332:string)  [unwired: 9 in, 1 out]
                n187 = Unbundle(w331) -> (w327:string[])
                n188 = Match First String(2:w327, 3:w332) -> (0:w328:i32)  [unwired: 1 out]
                n189 = property on="Ring" class="Ring (strict)"("Value"=w328, "Strings []"=w327) -> ()  [unwired: 2 in, 2 out]
                n190 = property on="Ring" class="Ring (strict)"("Visible"=TRUE) -> ()  [unwired: 2 in, 2 out]
                n191 = property on="Slider" class="Slide (strict)"("Visible"=FALSE) -> ()  [unwired: 2 in, 2 out]
              }
              frame Default {
                n192 = property on="Ring" class="Ring (strict)"("Visible"=FALSE) -> ()  [unwired: 2 in, 2 out]
                n193 = property on="Slider" class="Slide (strict)"("Visible"=FALSE) -> ()  [unwired: 2 in, 2 out]
              }
              frame "Brightness  **", "Color Level  **", "Compression  **", "FPS  **", "Sharpness  **" {
                n194 = call <vilib>:"NT Read Number.vi"("Name"=w339) -> ("Numeric"=w338:dbl)  [unwired: 9 in, 1 out]
                n195 = local write "Slider"(w338) -> ()
                n196 = property on="Slider" class="Slide (strict)"("Visible"=TRUE, "Scale.Maximum"=100.0 ("Scale.Range:Maximum")) -> ()  [unwired: 2 in, 2 out]
                n197 = property on="Ring" class="Ring (strict)"("Visible"=FALSE) -> ()  [unwired: 2 in, 2 out]
              }
            }
          }
        }
        n198 = property on="Progress" class="Clust (strict)"("Visible"=FALSE) -> ()  [unwired: 2 in, 2 out]
      }
      event "Test Name": Mouse Enter {
        # "Populate the ring with the list of tests"
        n199 = event-data() -> ()  [unwired: 1 in, 1 out]
        n200 = call <vilib>:"NT Read String Array.vi"("Name"="TestMode/TestList") -> ("String Array"=w346:string[])  [unwired: 9 in, 1 out]
        n201 = Build Array (concatenate)("Select the test to run...", w346) -> (w345:string[])
        n202 = property on="Test Name" class="Ring (strict)"("Strings []"=w345) -> ()  [unwired: 2 in, 2 out]
      }
      event "Test Name": Value Change {
        w348 = FALSE ("Visible")
        # "Tell the robot the test name to run"
        n203 = event-data() -> ("NewVal"=w352:u16)  [unwired: 1 in]
        n204 = property on="Test Name" class="Ring (strict)"() -> ("Strings []"=w353:string[])  [unwired: 2 in, 2 out]
        n205 = local write "Progress"(T5 {"Test Progress"=0, "Test Progress Text"=""} ("Progress")) -> ()
        n206 = Index Array(array=w353, index=w352) -> (element=w351:string)
        n207 = call <vilib>:"NT Write String.vi"("String"=w351, "Name"="TestMode/TestName") -> ()  [unwired: 9 in, 1 out]
        n208 = property on="Progress" class="Clust (strict)"("Visible"=TRUE) -> ()  [unwired: 2 in, 2 out]
        n209 = property on="Motor" class="Clust (strict)"("Visible"=w348) -> ()  [unwired: 2 in, 2 out]
        n210 = property on="Slider" class="Slide (strict)"("Visible"=w348) -> ()  [unwired: 2 in, 2 out]
        n211 = property on="On/Off" class="Bool (strict)"("Visible"=w348) -> ()  [unwired: 2 in, 2 out]
        n212 = property on="Rev/Fwd" class="Clust (strict)"("Visible"=w348) -> ()  [unwired: 2 in, 2 out]
        n213 = property on="Ring" class="Ring (strict)"("Visible"=w348) -> ()  [unwired: 2 in, 2 out]
      }
      event "Listbox": Double Click {
        n214 = event-data() -> ("PlatMods.Shift"=w356:bool, "Row"=w358:i32)  [unwired: 1 in]
        n215 = case shown="False" w356 {
          tunnel: w358 -> [w362 _]
          tunnel: 1 -> [w361 _]
          frame False {
            n216 = property on="Listbox" class="LstBox (strict)"() -> ("Item Symbols"=w360:i32[])  [unwired: 2 in, 2 out]
            n217 = Replace Array Subset(array=w360, new element=w361, index=w362) -> (w359:i32[])
            n218 = property on="Listbox" class="LstBox (strict)"("Item Symbols"=w359) -> ()  [unwired: 2 in, 2 out]
          }
          frame True {
            w363 = 0 ("Top Row")
            n219 = property on="Listbox" class="LstBox (strict)"() -> ("Number of Rows"=w365:u32)  [unwired: 2 in, 2 out]
            n220 = Initialize Array(0, w365) -> (w364:i32[])
            n221 = property on="Listbox" class="LstBox (strict)"("Top Row"=w363, "Value"=w363, "Item Symbols"=w364) -> ()  [unwired: 2 in, 2 out]
          }
        }
      }
      event "Listbox": Key Down {
        n222 = event-data() -> ("VKey"=w369:T19)  [unwired: 1 in]
        n223 = case shown="\"Left\", \"Right\"" w369 {
          selector: w369 -> [w374 _]
          tunnel: eventvkey."Left" ("VKey") -> [w372 _]
          frame "Left", "Right" {
            n224 = Equal?(x=w372, y=w374) -> (x = y?=w373:bool)
            n225 = Select(t=0, s=w373, f=1) -> (s? t:f=w375:i32)
            n226 = property on="Listbox" class="LstBox (strict)"() -> ("Item Symbols"=w378:i32[])  [unwired: 2 in, 2 out]
            n227 = Replace Array Subset(array=w378, new element=w375, index="Listbox") -> (w377:i32[])
            n228 = property on="Listbox" class="LstBox (strict)"("Item Symbols"=w377) -> ()  [unwired: 2 in, 2 out]
          }
          frame Default {
          }
        }
      }
      event "DB Camera Config": Value Change {
        n229 = event-data() -> ("NewVal"=w382:bool)  [unwired: 1 in]
        n230 = case shown="False" w382 {
          tunnel: w381 -> [w391 _]
          tunnel: [w384 w402] -> w380
          tunnel: w379 -> [w383 w402]
          frame False {
            w398 = "Camera"
            w401 = FALSE ("Visible")
            n231 = local read "Camera Settings"() -> (w390:T1)
            n232 = Index Array(array=w391) -> (element=w394:cluster{string[]})  [unwired: 1 in]
            n233 = Unbundle(w390) -> ("Frate Rate"=w389:i32, "Compression"=w388:i32, "Size"=w392:u16)
            n234 = Unbundle(w394) -> (w393:string[])
            n235 = Index Array(array=w393, index=w392) -> (element=w387:string)
            n236 = call-poly <vilib>:"Write Key.vi"("section"=w398, "value"=w387, "key"="Size", "refnum"=w383) -> ("refnum out"=w400:T18)  [unwired: 2 in, 5 out]
            n237 = call-poly <vilib>:"Write Key.vi"("section"=w398, "value"=w389, "key"="FrameRate", "refnum"=w400) -> ("refnum out"=w399:T18)  [unwired: 1 in, 6 out]
            n238 = property on="Camera Settings" class="Clust (strict)"("Visible"=w401) -> ()  [unwired: 2 in, 2 out]
            n239 = local write "DB Camera Config"(w401) -> ()
            n240 = call-poly <vilib>:"Write Key.vi"("section"=w398, "value"=w388, "key"="Compression", "refnum"=w399) -> ("refnum out"=w385:T18)  [unwired: 1 in, 6 out]
            n241 = call <vilib>:"Close Config Data.vi"("refnum"=w385) -> ("file path"=w386:path)  [unwired: 2 in, 8 out]
            n242 = call <vilib>:"Open Config Data.vi"("configuration file path"=w386) -> ("refnum"=w384:T18)  [unwired: 8 in, 2 out]
          }
          frame True {
            n243 = property on="Camera Settings" class="Clust (strict)"("Visible"=TRUE) -> ()  [unwired: 2 in, 2 out]
          }
        }
      }
      event "Camera Settings": Value Change {
        n244 = event-data() -> ("NewVal"=w415:T1)  [unwired: 1 in]
        n245 = Index Array(array=w411) -> (element=w410:cluster{string[]})  [unwired: 1 in]
        n246 = Unbundle(w415) -> ("Frate Rate"=w406:i32, "Compression"=w405:i32, "Size"=w408:u16)
        n247 = Unbundle(w410) -> (w409:string[])
        n248 = Index Array(array=w409, index=w408) -> (element=w407:string)
        n249 = Format Into String(format string="%s   %dfps   %d%%", w407, w406, w405) -> (resulting string=w412:string)  [unwired: 2 in, 1 out]
        n250 = Build Array(w412) -> (w413:string[])
        n251 = property on="DB Camera Config" class="Bool (strict)"("Strings [4]"=w413) -> ()  [unwired: 2 in, 2 out]
      }
      event "Motor.Enable": Value Change {
        n252 = event-data() -> ("NewVal"=w421:bool)  [unwired: 1 in]
        n253 = Unbundle("Motor") -> ("Value"=w420:dbl)  [unwired: 1 out]
        n254 = Select(t=w420, s=w421, f=0.0) -> (s? t:f=w418:dbl)
        n255 = call <vilib>:"NT Write Number.vi"("Numeric"=w418, "Name"=w417) -> ()  [unwired: 9 in, 1 out]
      }
      event "Slider": Value Change {
        n256 = event-data() -> ("NewVal"=w424:dbl)  [unwired: 1 in]
        n257 = call <vilib>:"NT Write Number.vi"("Numeric"=w424, "Name"=w425) -> ()  [unwired: 9 in, 1 out]
      }
      event "On/Off": Value Change {
        n258 = event-data() -> ("NewVal"=w429:bool)  [unwired: 1 in]
        n259 = Boolean To (0,1)(Boolean=w429) -> (0, 1=w428:i16)
        n260 = call <vilib>:"NT Write Number.vi"("Numeric"=w428, "Name"=w427) -> ()  [unwired: 9 in, 1 out]
      }
      event "Rev/Fwd": Value Change {
        n261 = event-data() -> ("NewVal.Forward"=w437:bool, "NewVal.Reverse"=w436:bool)  [unwired: 1 in]
        n262 = Boolean To (0,1)(Boolean=w437) -> (0, 1=w433:i16)
        n263 = Boolean To (0,1)(Boolean=w436) -> (0, 1=w435:i16)
        n264 = Negate(x=w435) -> (-x=w434:i16)
        n265 = Add(x=w433, y=w434) -> (x+y=w432:i16)
        n266 = call <vilib>:"NT Write Number.vi"("Numeric"=w432, "Name"=w431) -> ()  [unwired: 9 in, 1 out]
      }
      event "Ring": Value Change {
        n267 = event-data() -> ("NewVal"=w441:u16)  [unwired: 1 in]
        n268 = property on="Ring" class="Ring (strict)"() -> ("Strings []"=w442:string[])  [unwired: 2 in, 2 out]
        n269 = Index Array(array=w442, index=w441) -> (element=w440:string)
        n270 = call <vilib>:"NT Write String.vi"("String"=w440, "Name"=w439) -> ()  [unwired: 9 in, 1 out]
      }
    }
  }
  n271 = Index Array(array=w38) -> (element=w39:cluster{string[]})  [unwired: 1 in]
  n272 = Unbundle(w39) -> (w37:string[])
  n273 = Read from Text File(file (use dialog)=w15) -> (text=w14:string)  [unwired: 3 in, 3 out]
  n274 = Match Pattern(string=w14, regular expression="\\[Dev\\]") -> (before substring=w11:string, after substring=w12:string)  [unwired: 1 in, 2 out]
  n275 = local write "Dev Notes"(w12) -> ()
  n276 = local write "notes"(w11) -> ()
  n277 = Match First String(2:w37, 3:w36) -> (0:w35:i32)  [unwired: 1 out]
  n278 = Bundle("value"=w41, "value"=w40, "index"=w35) -> (w29:cluster{"value":i32, "value":i32, "index":i32})  [unwired: 1 out]
  n279 = while {
    tunnel: w15 -> [w445]
    stop <- FALSE stop-if-true
    n280 = local read "Dev Notes"() -> (w449:string)
    n281 = local read "notes"() -> (w444:string)
    n282 = feedback #1() -> (w443:string)  [unwired: 1 in]
    n283 = feedback-in #1(w449) -> ()
    n284 = feedback-in #2(w444) -> ()
    n285 = feedback #2() -> (w450:string)  [unwired: 1 in]
    n286 = Not Equal?(x=w449, y=w443) -> (x != y?=w447:bool)
    n287 = Not Equal?(x=w444, y=w450) -> (x != y?=w448:bool)
    n288 = Or(x=w448, y=w447) -> (x .or. y?=w446:bool)
    n289 = Wait (ms)(milliseconds to wait=1000) -> ()  [unwired: 1 out]
    n290 = case shown="True" w446 {
      tunnel: w445 -> [_ w457]
      tunnel: w444 -> [_ w455]
      tunnel: w443 -> [_ w454]
      frame False {
      }
      frame True {
        n291 = Concatenate Strings(w455, "[Dev]", w454) -> (w456:string)
        n292 = Write to Text File(file (use dialog)=w457, text=w456) -> ()  [unwired: 2 in, 3 out]
      }
    }
  }
  n293 = property on="On/Off" class="Bool (strict)"("Visible"=w52) -> ()  [unwired: 2 in, 2 out]
  n294 = property on="Motor" class="Clust (strict)"("Visible"=w52) -> ()  [unwired: 2 in, 2 out]
  n295 = property on="Progress" class="Clust (strict)"("Visible"=w52) -> ()  [unwired: 2 in, 2 out]
  n296 = property on="Ring" class="Ring (strict)"("Visible"=w52) -> ()  [unwired: 2 in, 2 out]
  n297 = property on="Camera Settings" class="Clust (strict)"("Val(Sgnl)"=w29) -> ()  [unwired: 2 in, 2 out]
  n298 = property on="Rev/Fwd" class="Clust (strict)"("Visible"=w52) -> ()  [unwired: 2 in, 2 out]
  n299 = property on="Camera Settings" class="Clust (strict)"("Visible"=w52) -> ()  [unwired: 2 in, 2 out]
  n300 = local write "DB Camera Config"(w52) -> ()
  "MotorName2" <- "Right Drive Motor"
  "MotorName1" <- "Left Drive Motor"
  "MotorName4" <- ""
  "MotorName3" <- "Arm Motor"
